vi "Retro Aspect Ratio Score 2015.vi"(10 "Aspect Fudge Factor":dbl=1.0, 11 "Rectangle Array ltrb":dbl[](array[numeric])=[2.22, 1.4]) -> (3 "Score":dbl)   [LabVIEW 2025]
doc: "Compare the ratio of the bounding box to that of the expected target. Score is in percent.\nFudge factor compensates for the cameras and camera modes that don't produce square pixels.\n\nSince inputs are particle measurements, the diagram doesn't expect to receive zero or negative values for either input."
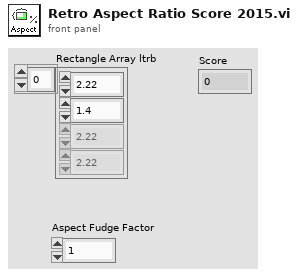
[diagram p1: front panel]
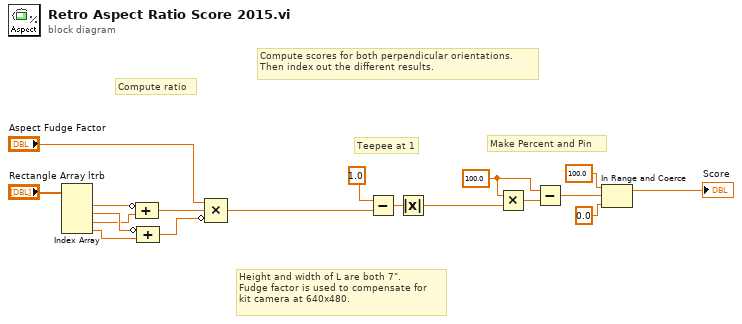
[diagram p0: block diagram]
diagram:
  w7 = 100.0 ("x/y")
  # "Make Percent and Pin"
  # "Teepee at 1"
  # "Height and width of L are both 7\".\nFudge factor is used to compensate for\nkit camera at 640x480."
  # "Compute scores for both perpendicular orientations.\nThen index out the different results."
  # "Compute ratio"
  n1 = Index Array(array="Rectangle Array ltrb") -> (element #1=w15:dbl, element #2=w18:dbl, element #3=w16:dbl, element #4=w17:dbl)  [unwired: 4 in]
  n2 = Compound Arithmetic op=ADD(invert w15, w16) -> (w14:dbl)
  n3 = Compound Arithmetic op=ADD(invert w18, w17) -> (w13:dbl)
  n4 = Compound Arithmetic op=MULTIPLY("Aspect Fudge Factor", w14, invert w13) -> (w1:dbl)
  n5 = Subtract(x=1.0 ("y"), y=w1) -> (x-y=w5:dbl)
  n6 = Absolute Value(x=w5) -> (abs(x)=w8:dbl)
  n7 = Multiply(x=w7, y=w8) -> (x*y=w9:dbl)
  n8 = Subtract(x=w7, y=w9) -> (x-y=w4:dbl)
  n9 = In Range and Coerce(upper limit=100.0, x=w4, lower limit=0.0) -> (coerced(x)=→"Score":dbl)  [unwired: 1 out]
